vi "ServoController_init.vi"(8 "Error In":errorcluster, 11 "Servo Controller Index":u8) -> (0 "Error Out":errorcluster)   [LabVIEW 2013]
uses:
  <vilib>/myRIO/Instrument Drivers/Onboard IO/I2C/vis/Smart Open.vi
  <vilib>/myRIO/Instrument Drivers/Onboard IO/I2C/vis/Configure.vi
  <vilib>/myRIO/Instrument Drivers/Onboard IO/I2C/vis/Write.vi
  <vilib>/myRIO/Instrument Drivers/Onboard IO/I2C/vis/Write Read.vi
  <vilib>/myRIO/Instrument Drivers/Onboard IO/I2C/vis/Open.vi
  <vilib>/myRIO/Common/Instrument Driver Framework/myRIO v1.0/I2C/vis/myRIO v1.1 Open I2C.vi
  <vilib>/myRIO/Common/Instrument Driver Framework/Utilities/vis/Validate Channels.vi
  <vilib>/myRIO/Common/Instrument Driver Framework/myRIO v1.0/I2C/vis/myRIO v1.0 Reserve I2C.vi
  <vilib>/myRIO/Common/Instrument Driver Framework/myRIO v1.0/I2C/vis/myRIO v1.0 Build MUX Configuration I2C.vi
  <vilib>/myRIO/Common/Instrument Driver Framework/myRIO v1.0/Resource Manager/vis/myRIO v1.0 Reserve Channel List.vi
  <vilib>/myRIO/Common/Instrument Driver Framework/myRIO v1.0/Resource Manager/vis/myRIO v1.0 Create Configuration List.vi
  <vilib>/myRIO/Common/Instrument Driver Framework/myRIO v1.0/Resource Manager/vis/myRIO v1.0 Reserve Channel.vi
  <vilib>/myRIO/Common/Instrument Driver Framework/myRIO v1.0/Resource Manager/vis/myRIO v1.0 Unreserve Channel.vi
  <vilib>/myRIO/Common/Instrument Driver Framework/myRIO v1.0/Resource Manager/vis/myRIO v1.0 Build Mutex Name.vi
  <vilib>/myRIO/Common/Instrument Driver Framework/myRIO v1.0/myRIO v1.1 Open.vi
  <vilib>/Utility/VariantDataType/GetNumericInfo.vi
  <vilib>/Utility/error.llb/Error Cluster From Error Code.vi
  <vilib>/myRIO/Common/Instrument Driver Framework/Utilities/vis/IO Manager.vi
  <vilib>/myRIO/Common/Instrument Driver Framework/Utilities/vis/Configuration Manager.vi
  <vilib>/myRIO/Common/Instrument Driver Framework/myRIO v1.0/Resource Manager/vis/myRIO v1.0 Configure IO.vi
  <vilib>/myRIO/Common/Instrument Driver Framework/myRIO v1.0/myRIO v1.0 Close.vi
  <vilib>/myRIO/Common/Instrument Driver Framework/myRIO v1.0/I2C/vis/myRIO v1.0 Configure I2C.vi
  <vilib>/myRIO/Common/Instrument Driver Framework/myRIO v1.0/I2C/vis/myRIO v1.0 Write I2C.vi
  <vilib>/myRIO/Common/Instrument Driver Framework/myRIO v1.0/I2C/vis/myRIO v1.0 Read I2C.vi
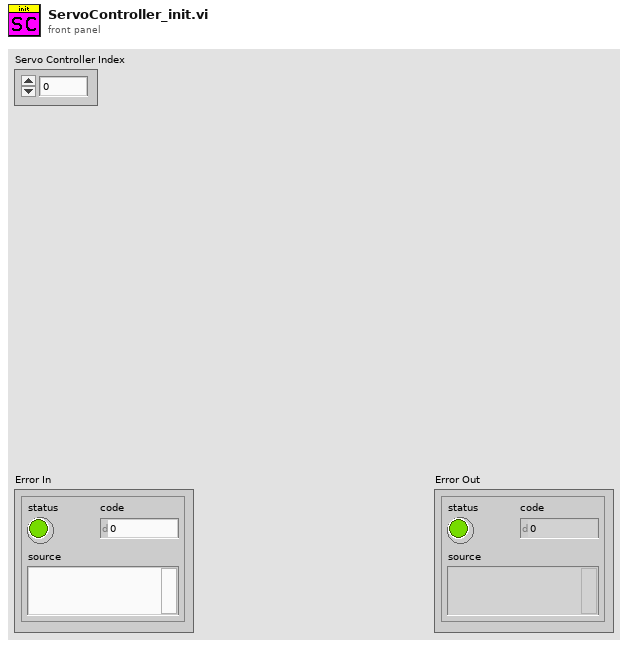
[diagram p1: front panel]
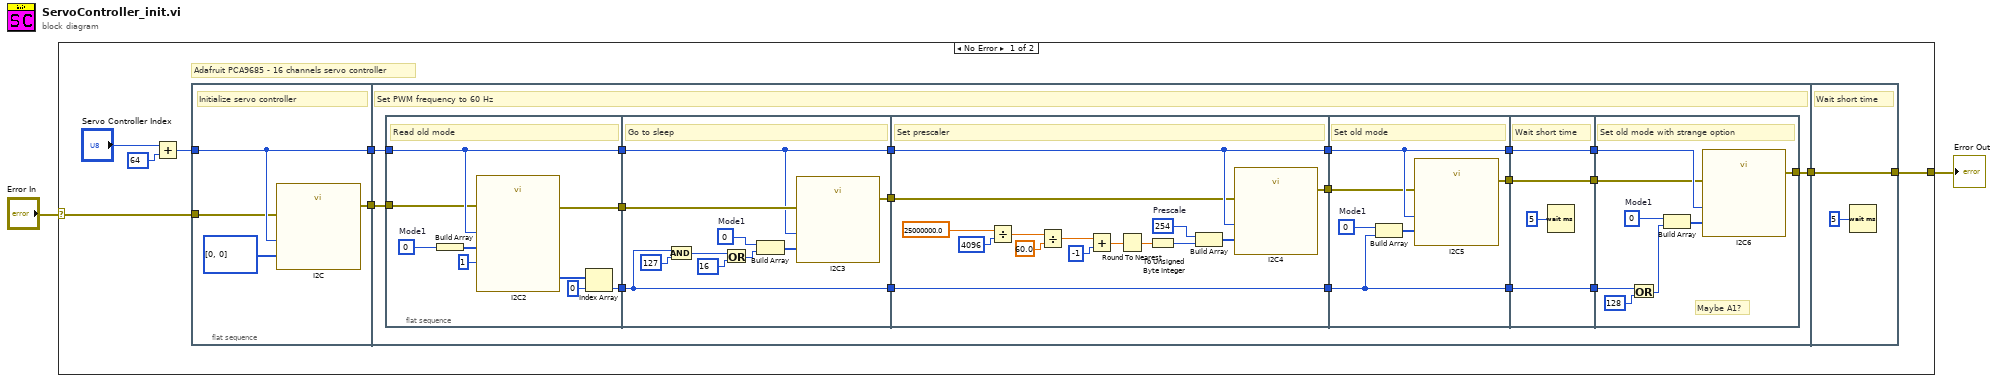
[diagram p0: block diagram]
diagram:
  n1 = case shown="No Error" "Error In" {
    selector: "Error In" -> [w3 w87]
    tunnel: [w4 w87] -> w2
    frame No Error {
      # "Adafruit PCA9685 - 16 channels servo controller"
      n2 = Add(x="Servo Controller Index", y=u8 64 ("Slave Address (7-bit)")) -> (x+y=w6:u8)
      n3 = flat-sequence {
        tunnel: w6 -> [w13]
        tunnel: [w13] -> w10
        tunnel: [w12] -> w9
        tunnel: w3 -> [w11]
        tunnel: w10 -> [w32]
        tunnel: w9 -> [w29]
        tunnel: [w15] -> w8
        tunnel: [w86] -> w4
        tunnel: w8 -> [w86]
        frame #0 {
          # "Initialize servo controller"
          n4 = call "I2C"("Slave Address (7-bit)"=w13, "Bytes to Write"=u8[] [0, 0], "error in (no error)"=w11) -> ("error out"=w12:errorcluster)  [unwired: 24 in]
        }
        frame #1 {
          # "Set PWM frequency to 60 Hz"
          n5 = flat-sequence {
            tunnel: w32 -> [w39]
            tunnel: [w39] -> w31
            tunnel: [w38] -> w30
            tunnel: w29 -> [w37]
            tunnel: [w36] -> w28
            tunnel: w31 -> [w44]
            tunnel: w30 -> [w50]
            tunnel: w28 -> [w45]
            tunnel: [w45] -> w27
            tunnel: [w44] -> w26
            tunnel: [w43] -> w16
            tunnel: w27 -> [w65]
            tunnel: w26 -> [w63]
            tunnel: [w65] -> w25
            tunnel: [w63] -> w24
            tunnel: [w53] -> w17
            tunnel: w16 -> [w52]
            tunnel: w25 -> [w71]
            tunnel: w24 -> [w70]
            tunnel: [w71] -> w22
            tunnel: [w70] -> w21
            tunnel: [w69] -> w19
            tunnel: w17 -> [w68]
            tunnel: [w75] -> w23
            tunnel: w22 -> [w75]
            tunnel: w21 -> [w74]
            tunnel: [w74] -> w20
            tunnel: w19 -> [w73]
            tunnel: [w73] -> w18
            tunnel: w23 -> [w83]
            tunnel: w20 -> [w80]
            tunnel: w18 -> [w79]
            tunnel: [w78] -> w15
            frame #0 {
              w34 = u8 0  # Mode1
              # "Read old mode"
              n6 = Build Array(w34) -> (w33:u8[])
              n7 = call "I2C2"("Slave Address (7-bit)"=w39, "Bytes to Write"=w33, "Byte Count"=u32 1, "error in (no error)"=w37) -> ("Bytes Read"=w40:u8[], "error out"=w38:errorcluster)  [unwired: 22 in]
              n8 = Index Array(array=w40, index=0) -> (element=w36:u8)
            }
            frame #1 {
              w51 = u8 0  # Mode1
              # "Go to sleep"
              n9 = And(x=w45, y=u8 127 ("Slave Address (7-bit)")) -> (x .and. y?=w49:u8)
              n10 = Or(x=w49, y=u8 16 ("Slave Address (7-bit)")) -> (x .or. y?=w47:u8)
              n11 = Build Array(w51, w47) -> (w42:u8[])
              n12 = call "I2C3"("Slave Address (7-bit)"=w44, "Bytes to Write"=w42, "error in (no error)"=w50) -> ("error out"=w43:errorcluster)  [unwired: 24 in]
            }
            frame #2 {
              w66 = u8 254  # Prescale
              # "Set prescaler"
              n13 = Divide(x=25000000.0, y=4096) -> (x/y=w57:dbl)
              n14 = Divide(x=w57, y=60.0) -> (x/y=w55:dbl)
              n15 = Add(x=w55, y=-1) -> (x+y=w59:dbl)
              n16 = Round To Nearest(number=w59) -> (nearest integer value=w58:dbl)
              n17 = To Unsigned Byte Integer(number=w58) -> (unsigned 8bit integer=w54:u8)
              n18 = Build Array(w66, w54) -> (w64:u8[])
              n19 = call "I2C4"("Slave Address (7-bit)"=w63, "Bytes to Write"=w64, "error in (no error)"=w52) -> ("error out"=w53:errorcluster)  [unwired: 24 in]
            }
            frame #3 {
              w72 = u8 0  # Mode1
              # "Set old mode"
              n20 = Build Array(w72, w71) -> (w67:u8[])
              n21 = call "I2C5"("Slave Address (7-bit)"=w70, "Bytes to Write"=w67, "error in (no error)"=w68) -> ("error out"=w69:errorcluster)  [unwired: 24 in]
            }
            frame #4 {
              # "Wait short time"
              n22 = Wait (ms)(milliseconds to wait=u32 5) -> ()  [unwired: 1 out]
            }
            frame #5 {
              w84 = u8 0  # Mode1
              # "Maybe A1?"
              # "Set old mode with strange option"
              n23 = Or(x=w83, y=u8 128 ("Slave Address (7-bit)")) -> (x .or. y?=w81:u8)
              n24 = Build Array(w84, w81) -> (w77:u8[])
              n25 = call "I2C6"("Slave Address (7-bit)"=w80, "Bytes to Write"=w77, "error in (no error)"=w79) -> ("error out"=w78:errorcluster)  [unwired: 24 in]
            }
          }
        }
        frame #2 {
          # "Wait short time"
          n26 = Wait (ms)(milliseconds to wait=u32 5) -> ()  [unwired: 1 out]
        }
      }
    }
    frame Error {
    }
  }
  "Error Out" <- w2
